vi "addServer.vi"(6 "TypeString in":string, 8 "error in (no error)":errorcluster, 9 "Server in":refnum<class "IServer.lvclass">, 10 "ServerConfig in":refnum<class "IPropertyObject.lvclass">, 11 "IDevice in":refnum<class "IDevice.lvclass">) -> (0 "error out":errorcluster, 1 "Server out":refnum<class "IServer.lvclass">, 2 "ServerConfig out":refnum<class "IPropertyObject.lvclass">, 3 "IDevice out":refnum<class "IDevice.lvclass">)   [LabVIEW 2022 SP3, in "openDAQ.lvlib" / "IBaseObject.lvlib" / "IPropertyObject.lvlib" / "IComponent.lvlib" / "IFolder.lvlib" / "IDevice.lvlib" / "IDevice.lvclass"]
uses:
  <instrlib>/openDAQ/Public/Classes/IDevice/IDevice.lvclass
  C:/Program Files (x86)/National Instruments/LabVIEW 2022/instr.lib/openDAQ/Public/Classes/IBaseObject/IBaseObject.lvclass
  <instrlib>/openDAQ/Public/Classes/IPropertyObject/IPropertyObject.lvclass
  <instrlib>/openDAQ/Public/Classes/IServer/IServer.lvclass
  <instrlib>/openDAQ/Public/Classes/IBaseObject/IBaseObject.lvclass/IBaseObject.ctl
  <instrlib>/openDAQ/Public/Classes/IBaseObject/Accessor/Read reference.vi
  <instrlib>/openDAQ/Public/Classes/IBaseObject/Accessor/Write reference.vi
  <instrlib>/openDAQ/Public/Classes/daqCoreTypes/IString/IString.lvclass
  <instrlib>/openDAQ/Binaries/Windows/x86/copendaq32.dll
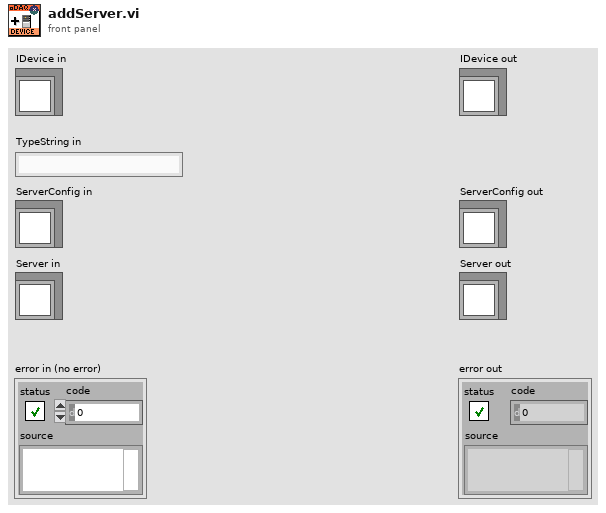
[diagram p1: front panel]
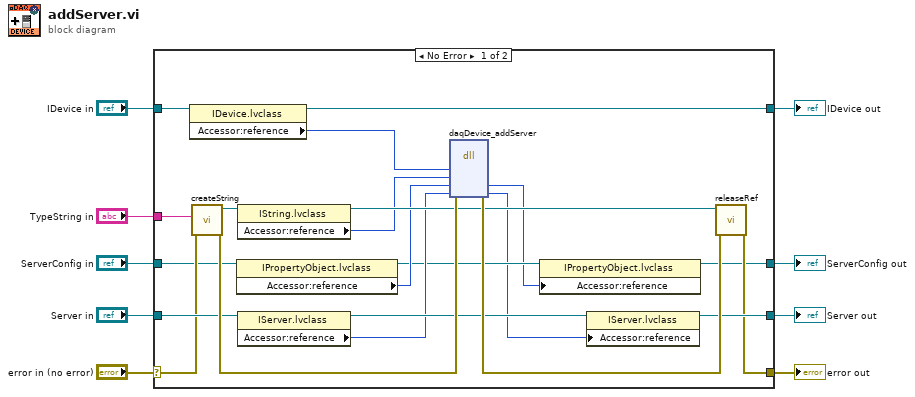
[diagram p0: block diagram]
diagram:
  n1 = case shown="No Error" "error in (no error)" {
    selector: "error in (no error)" -> [w21 w34]
    tunnel: [w18 w34] -> w8
    tunnel: [w26 w33] -> w6
    tunnel: "IDevice in" -> [w27 w33]
    tunnel: "Server in" -> [w25 w32]
    tunnel: [w24 w32] -> w2
    tunnel: "TypeString in" -> [w22 _]
    tunnel: "ServerConfig in" -> [w17 w31]
    tunnel: [w10 w31] -> w1
    frame No Error {
      n2 = property class="IDevice.lvclass"(reference=w27) -> (reference out=w26:refnum<class "IDevice.lvclass">, "Accessor:reference"=w23:i64)  [unwired: 1 in, 1 out]
      n3 = call <instrlib>:"createString.vi"("error in (no error)"=w21, "String"=w22) -> ("error out"=w30:errorcluster, "IString out"=w20:refnum<class "IString.lvclass">)  [unwired: 8 in]
      n4 = property class="IPropertyObject.lvclass"(reference=w17) -> (reference out=w13:refnum<class "IPropertyObject.lvclass">, "Accessor:reference"=w15:i64)  [unwired: 1 in, 1 out]
      n5 = property class="IString.lvclass"(reference=w20) -> (reference out=w19:refnum<class "IString.lvclass">, "Accessor:reference"=w16:i64)  [unwired: 1 in, 1 out]
      n6 = property class="IServer.lvclass"(reference=w25) -> (reference out=w28:refnum<class "IServer.lvclass">, "Accessor:reference"=w14:i64)  [unwired: 1 in, 1 out]
      n7 = dll-call lib="C:/Program Files (x86)/National Instruments/LabVIEW 2022/instr.lib/openDAQ/Binaries/Windows/x86/copendaq*.*" fn="daqDevice_addServer"(error in=w30, "device"=w23, "typeStr"=w16, "serverConfig"=w15, "server"=w14) -> (error out=w29:errorcluster, "serverConfig"=w12:i64, "server"=w11:i64)  [unwired: 5 in, 1 out]
      n8 = property class="IPropertyObject.lvclass"(reference=w13, "Accessor:reference"=w12) -> (reference out=w10:refnum<class "IPropertyObject.lvclass">)  [unwired: 1 in, 1 out]
      n9 = property class="IServer.lvclass"(reference=w28, "Accessor:reference"=w11) -> (reference out=w24:refnum<class "IServer.lvclass">)  [unwired: 1 in, 1 out]
      n10 = call-dynamic "releaseRef.vi"("error in (no error)"=w29, "IBaseObject in"=w19) -> ("error out"=w18:errorcluster)  [unwired: 9 in]
    }
    frame Error {
    }
  }
  "error out" <- w8
  "IDevice out" <- w6
  "Server out" <- w2
  "ServerConfig out" <- w1
